vi "3-2.vi"() -> ()   [LabVIEW 2019, in "AoC2022.lvlib"]
uses:
  AoC2022.lvlib
panel:
  out "Numeric":i32
  out "string 3":string
  out "sum":u32
  out "string 2":string
  out "string":string
  out "Array":u8[](array[numeric])
  out "subarray 2":u8[](array[numeric])
  out "subarray":u8[](array[numeric])
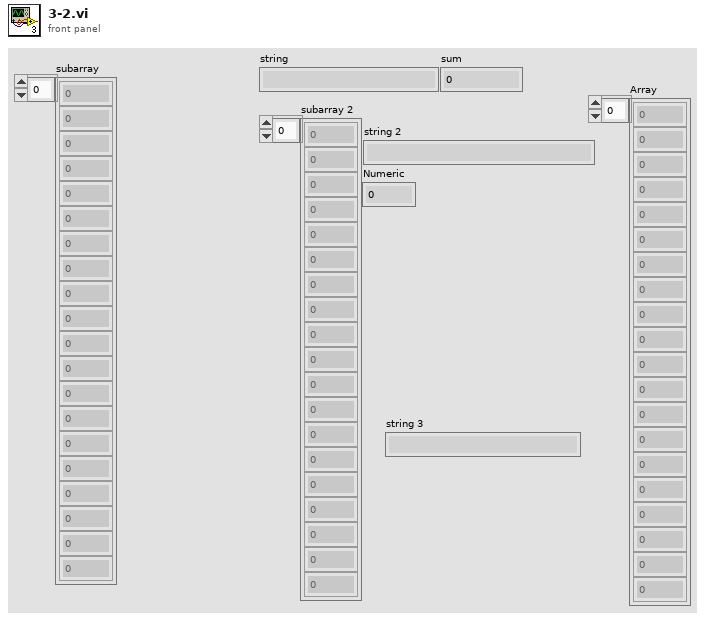
[diagram p1: front panel]
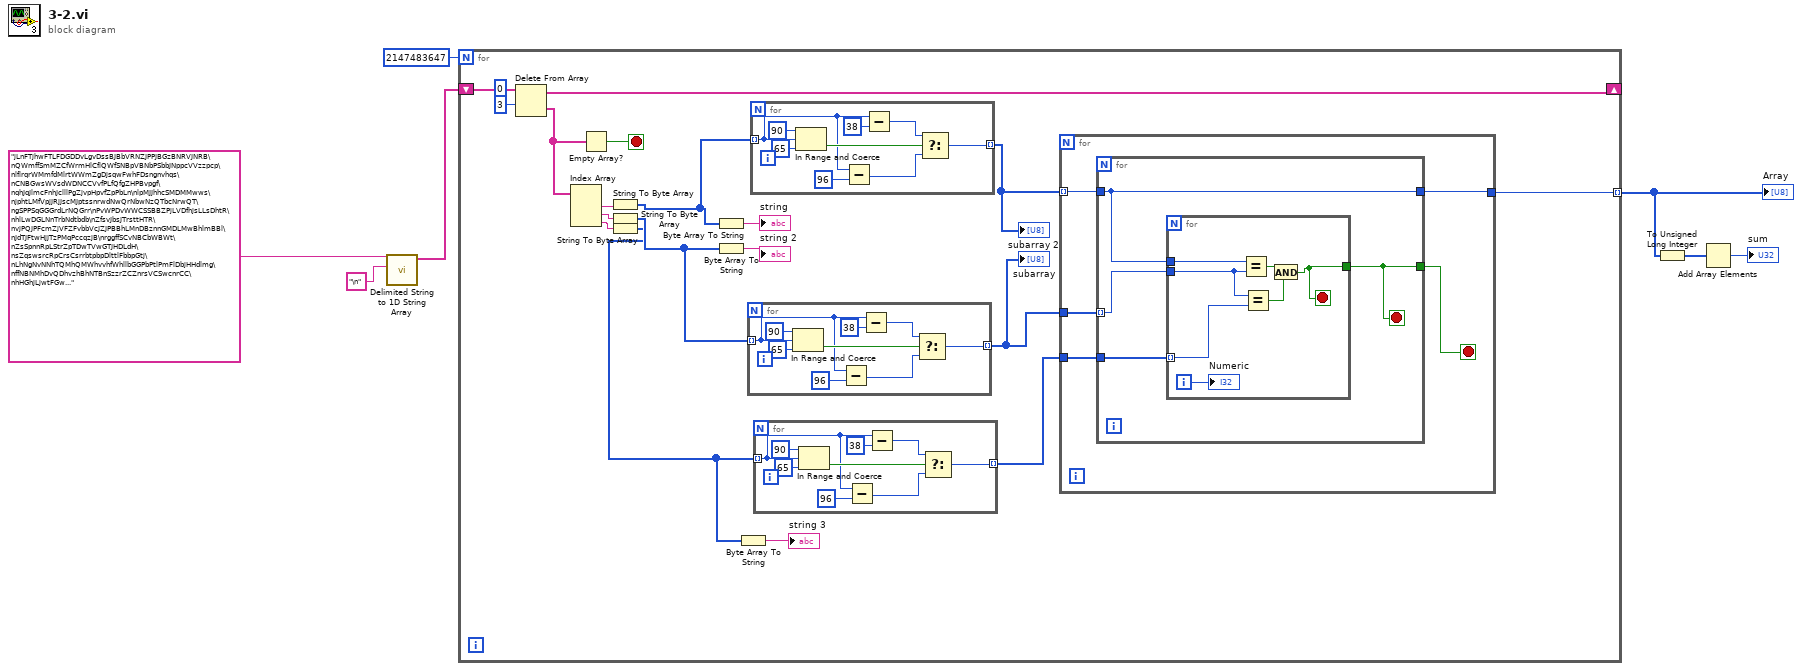
[diagram p0: block diagram]
diagram:
  n1 = call <vilib>:"Delimited String to 1D String Array.vi"("delimiter"="\n", "delimited string"="jLnFTjhwFTLFDGDDvLgvDssBJBbVRNZJPPJBGzBNRVJNRB\nQWmffSmMZCfWrmHlCflQWfSNBpVBNbPSbbJNppcVVzzpcp\nlflrqrWMmfdMlrtWWmZgDjsqwFwhFDsngnvhqs\nCNBGwsWVsdWDNCCVvfPLfQfgZHPBvpgf\nqhJqJlmcFnhJclllPgZjvpHpvfZpPbLn\nlpMJJhhcSMDMMwws\njphtLMfVpjJRjJscMJptssnrwdNwQrNbwNzQTbcNrwQT\ngSPPSqGGGrdLrNQGrr\nPvWPDvWWCSSBBZPjLVDfhjsLLsDhtR\nhlLwDGLNnTrbNdtbdb\nZfsvJbsJTrsttHTR\nvjPQJPFcmZjVFZFvbbVcJZJPBBhLMnDBznnGMDLMwBhlmBBl\nJdTJFtwHjJTzPMqPccqzjB\nrggffSCvNBCbWBWt\nZsSpnnRpLStrZpTDwTVwGTJHDLdH\nsZqswsrcRpCrsCsrrbtpbpDlttlFbbpGtj\nLhNgNvNNhTQMhQMWhvvhfWhllbGGPbPtlPmFlDbjHHdlmg\nffNBNMhDvQDhvzhBhNTBnSzzrZCZnrsVCSwcnrCC\nhHGhjLjwtFGw...") -> ("string array"=w2:string[])  [unwired: 9 in]
  n2 = for {
    N: 2147483647 -> [_]
    tunnel: [w26] -> w5 mode=indexing
    shift-right: [w20] -> _
    shift-left: w2 -> [w21]
    stop <- w11 stop-if-true
    n3 = Delete From Array(array=w21, length=3, index=0) -> (deleted portion=w17:string[], array with subset deleted=w20:string[])
    n4 = Index Array(array=w17) -> (element #1=w16:string, element #2=w15:string, element #3=w14:string)  [unwired: 3 in]
    n5 = Empty Array?(array=w17) -> (empty?=w11:bool)
    n6 = String To Byte Array(string=w16) -> (unsigned byte array=w13:u8[])
    n7 = String To Byte Array(string=w15) -> (unsigned byte array=w12:u8[])
    n8 = String To Byte Array(string=w14) -> (unsigned byte array=w9:u8[])
    n9 = Byte Array To String(unsigned byte array=w13) -> (string=→"string":string)
    n10 = Byte Array To String(unsigned byte array=w12) -> (string=→"string 2":string)
    n11 = Byte Array To String(unsigned byte array=w9) -> (string=→"string 3":string)
    n12 = for {
      tunnel: w12 -> [w52] mode=indexing
      tunnel: [w55] -> w24 mode=indexing
      n13 = In Range and Coerce(upper limit=u8 90, x=w52, lower limit=u8 65) -> (In Range?=w58:bool)  [unwired: 1 out]
      n14 = Subtract(x=w52, y=u8 96) -> (x-y=w53:u8)
      n15 = Subtract(x=w52, y=u8 38) -> (x-y=w56:u8)
      n16 = Select(t=w56, s=w58, f=w53) -> (s? t:f=w55:u8)
    }
    "subarray" <- w24
    n17 = for {
      tunnel: w13 -> [w61] mode=indexing
      tunnel: [w64] -> w25 mode=indexing
      n18 = In Range and Coerce(upper limit=u8 90, x=w61, lower limit=u8 65) -> (In Range?=w67:bool)  [unwired: 1 out]
      n19 = Subtract(x=w61, y=u8 96) -> (x-y=w62:u8)
      n20 = Subtract(x=w61, y=u8 38) -> (x-y=w65:u8)
      n21 = Select(t=w65, s=w67, f=w62) -> (s? t:f=w64:u8)
    }
    "subarray 2" <- w25
    n22 = for {
      tunnel: w9 -> [w27] mode=indexing
      tunnel: [w30] -> w8 mode=indexing
      n23 = In Range and Coerce(upper limit=u8 90, x=w27, lower limit=u8 65) -> (In Range?=w33:bool)  [unwired: 1 out]
      n24 = Subtract(x=w27, y=u8 96) -> (x-y=w28:u8)
      n25 = Subtract(x=w27, y=u8 38) -> (x-y=w31:u8)
      n26 = Select(t=w31, s=w33, f=w28) -> (s? t:f=w30:u8)
    }
    n27 = for {
      tunnel: w25 -> [w39] mode=indexing
      tunnel: w24 -> [w40]
      tunnel: [w37] -> w26
      tunnel: w8 -> [w36]
      stop <- w38 stop-if-true
      n28 = for {
        tunnel: w40 -> [w44] mode=indexing
        tunnel: w39 -> [w42]
        tunnel: [w43] -> w38
        tunnel: [w42] -> w37
        tunnel: w36 -> [w41]
        stop <- w43 stop-if-true
        n29 = for {
          tunnel: w44 -> [w50]
          tunnel: [w46] -> w43
          tunnel: w42 -> [w51]
          tunnel: w41 -> [w49] mode=indexing
          i -> [w45]
          stop <- w46 stop-if-true
          n30 = Equal?(x=w51, y=w50) -> (x = y?=w48:bool)
          n31 = Equal?(x=w50, y=w49) -> (x = y?=w47:bool)
          n32 = And(x=w48, y=w47) -> (x .and. y?=w46:bool)
          "Numeric" <- w45
        }
      }
    }
  }
  "Array" <- w5
  n33 = To Unsigned Long Integer(number=w5) -> (unsigned 32bit integer=w4:u32[])
  n34 = Add Array Elements(numeric array=w4) -> (sum=→"sum":u32)
